vi "RSNRPZ Get ContAv Aperture.vi"(8 "error in (no error)":errorcluster, 10 "Channel (1)":i32=1, 11 "VISA session":refnum<visa-resource-name> caption="VISA resource name") -> (0 "error out":errorcluster, 2 "ContAv Aperture":dbl format="%.2p", 3 "dup VISA session":refnum<visa-resource-name> caption="VISA resource name")   [LabVIEW 2010]
doc: "This VI queries the value of ContAv mode aperture size.\n\nRemote-control command(s):\nSENS:POW:AVG:APER?"
uses:
  rsnrpz_32.dll
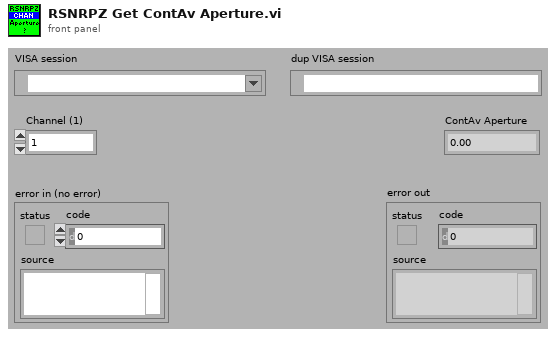
[diagram p1: front panel]
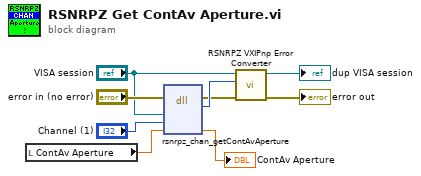
[diagram p0: block diagram]
diagram:
  n1 = local read "ContAv Aperture"() -> (w7:dbl)
  n2 = dll-call lib="rsnrpz_32.dll" fn="rsnrpz_chan_getContAvAperture"(error in="error in (no error)", "VISA Session"="VISA session", "Channel"="Channel (1)", "ContAv Aperture"=w7) -> (error out=w5:errorcluster, "Status"=w9:i32, "ContAv Aperture"=→"ContAv Aperture":dbl)  [unwired: 4 in, 1 out]
  n3 = call <instrlib>:"RSNRPZ VXIPnp Error Converter.vi"("error in"=w5, "VXIPnp error code"=w9, "VISA session"="VISA session") -> ("error out"=→"error out":errorcluster, "dup VISA session"=→"dup VISA session":refnum<visa-resource-name>)  [unwired: 7 in]
